vi "Autonomous Independent.vi"() -> ()   [LabVIEW 2015]
doc: "This VI is called when autonomous begins, and will automatically be terminated when autonomous ends. You can carry out timed or sensor driven robot movement independently without needing to return to the caller."
uses:
  <vilib>/Rock Robotics/WPI/SafetyOutput/WPI_SafetyOutputConfigMenu.ctl
  <vilib>/Rock Robotics/Network Tables/NT Read Number.vi
  <vilib>/Rock Robotics/WPI/Utilities/WPI_GetSetVariantRefNum.vi
  <vilib>/Rock Robotics/WPI/Solenoid/Deprecated/WPI_SolenoidGetBool.vi
  <vilib>/Rock Robotics/WPI/Solenoid/Deprecated/WPI_SolenoidSetBool.vi
panel:
  out "Defense Type":dbl=6.0
  in  "Auton_Modes":T1(array[cluster])=[{"Actions"=[{"Action"=enum."Drive", "Effort"=0.55, "Duration"=3.5}, {"Action"=enum."Nothing", "Effort"=0.0, "Duration"=0.0}]}, {"Actions"=[{"Action"=enum."Art Down", "Effort"=0.0, "Duration"=1.0}, {"Action"=enum."Drive", "Effort"=0.75, "Duration"=5.0}, {"Action"=enum."Art Up", "Effort"=0.0, "Duration"=1.0}]}, {"Actions"=[{"Action"=enum."Drive", "Effort"=1.0, "Duration"=3.0}, {"Action"=enum."Art Down", "Effort"=0.0, "Duration"=1.0}, {"Action"=enum."Drive", "Effort"=0.75, "Duration"=3.5}, {"Action"=enum."Art Up", "Effort"=0.0, "Duration"=1.0}]}, {"Actions"=[{"Action"=enum."Shift", "Effort"=0.5, "Duration"=0.0}, {"Action"=enum."Drive", "Effort"=1.0, "Duration"=0.1}, {"Action"=enum."Nothing", "Effort"=0.0, "Duration"=0.1}, {"Action"=enum."Drive", "Effort"=1.0, "Duration"=3.0}]}, {"Actions"=[{"Action"=enum."Shift", "Effort"=0.0, "Duration"=0.0}, {"Action"=enum."Drive", "Effort"=1.0, "Duration"=0.1}, {"Action"=enum."Nothing", "Effort"=0.0, "Duration"=0.1}, {"Action"=enum."Drive", "Effort"=1.0, "Duration"=3.0}]}, {"Actions"=[{"Action"=enum."Shift", "Effort"=0.0, "Duration"=0.0}, {"Action"=enum."Drive", "Effort"=1.0, "Duration"=0.1}, {"Action"=enum."Nothing", "Effort"=0.0, "Duration"=0.1}, {"Action"=enum."Drive", "Effort"=1.0, "Duration"=3.0}]}, {"Actions"=[{"Action"=enum."Drive", "Effort"=0.55, "Duration"=4.0}, {"Action"=enum."Art Down", "Effort"=0.0, "Duration"=1.0}, {"Action"=enum."Drive", "Effort"=-0.5, "Duration"=0.5}, {"Action"=enum."Drive", "Effort"=0.75, "Duration"=1.0}, {"Action"=enum."Art Up", "Effort"=0.0, "Duration"=1.0}, {"Action"=enum."Drive", "Effort"=0.75, "Duration"=3.0}]}, {"Actions"=[{"Action"=enum."Art Down", "Effort"=0.0, "Duration"=0.5}, {"Action"=enum."Drive", "Effort"=0.55, "Duration"=4.25}, {"Action"=enum."Art Up", "Effort"=0.0, "Duration"=0.0}, {"Action"=enum."Nothing", "Effort"=0.0, "Duration"=0.3}, {"Action"=enum."Drive", "Effort"=0.9, "Duration"=2.0}]}, {"Actions"=[{"Action"=enum."Nothing", "Effort"=0.0, "Duration"=0.0}]}]
  # "0 Reach Defense\n1 Low Bar\n2 Rough Terrain\n3 Moat\n4 Rock Wall\n5 Ramparts\n6 Cheval\n7 Portcullis\n8 None"
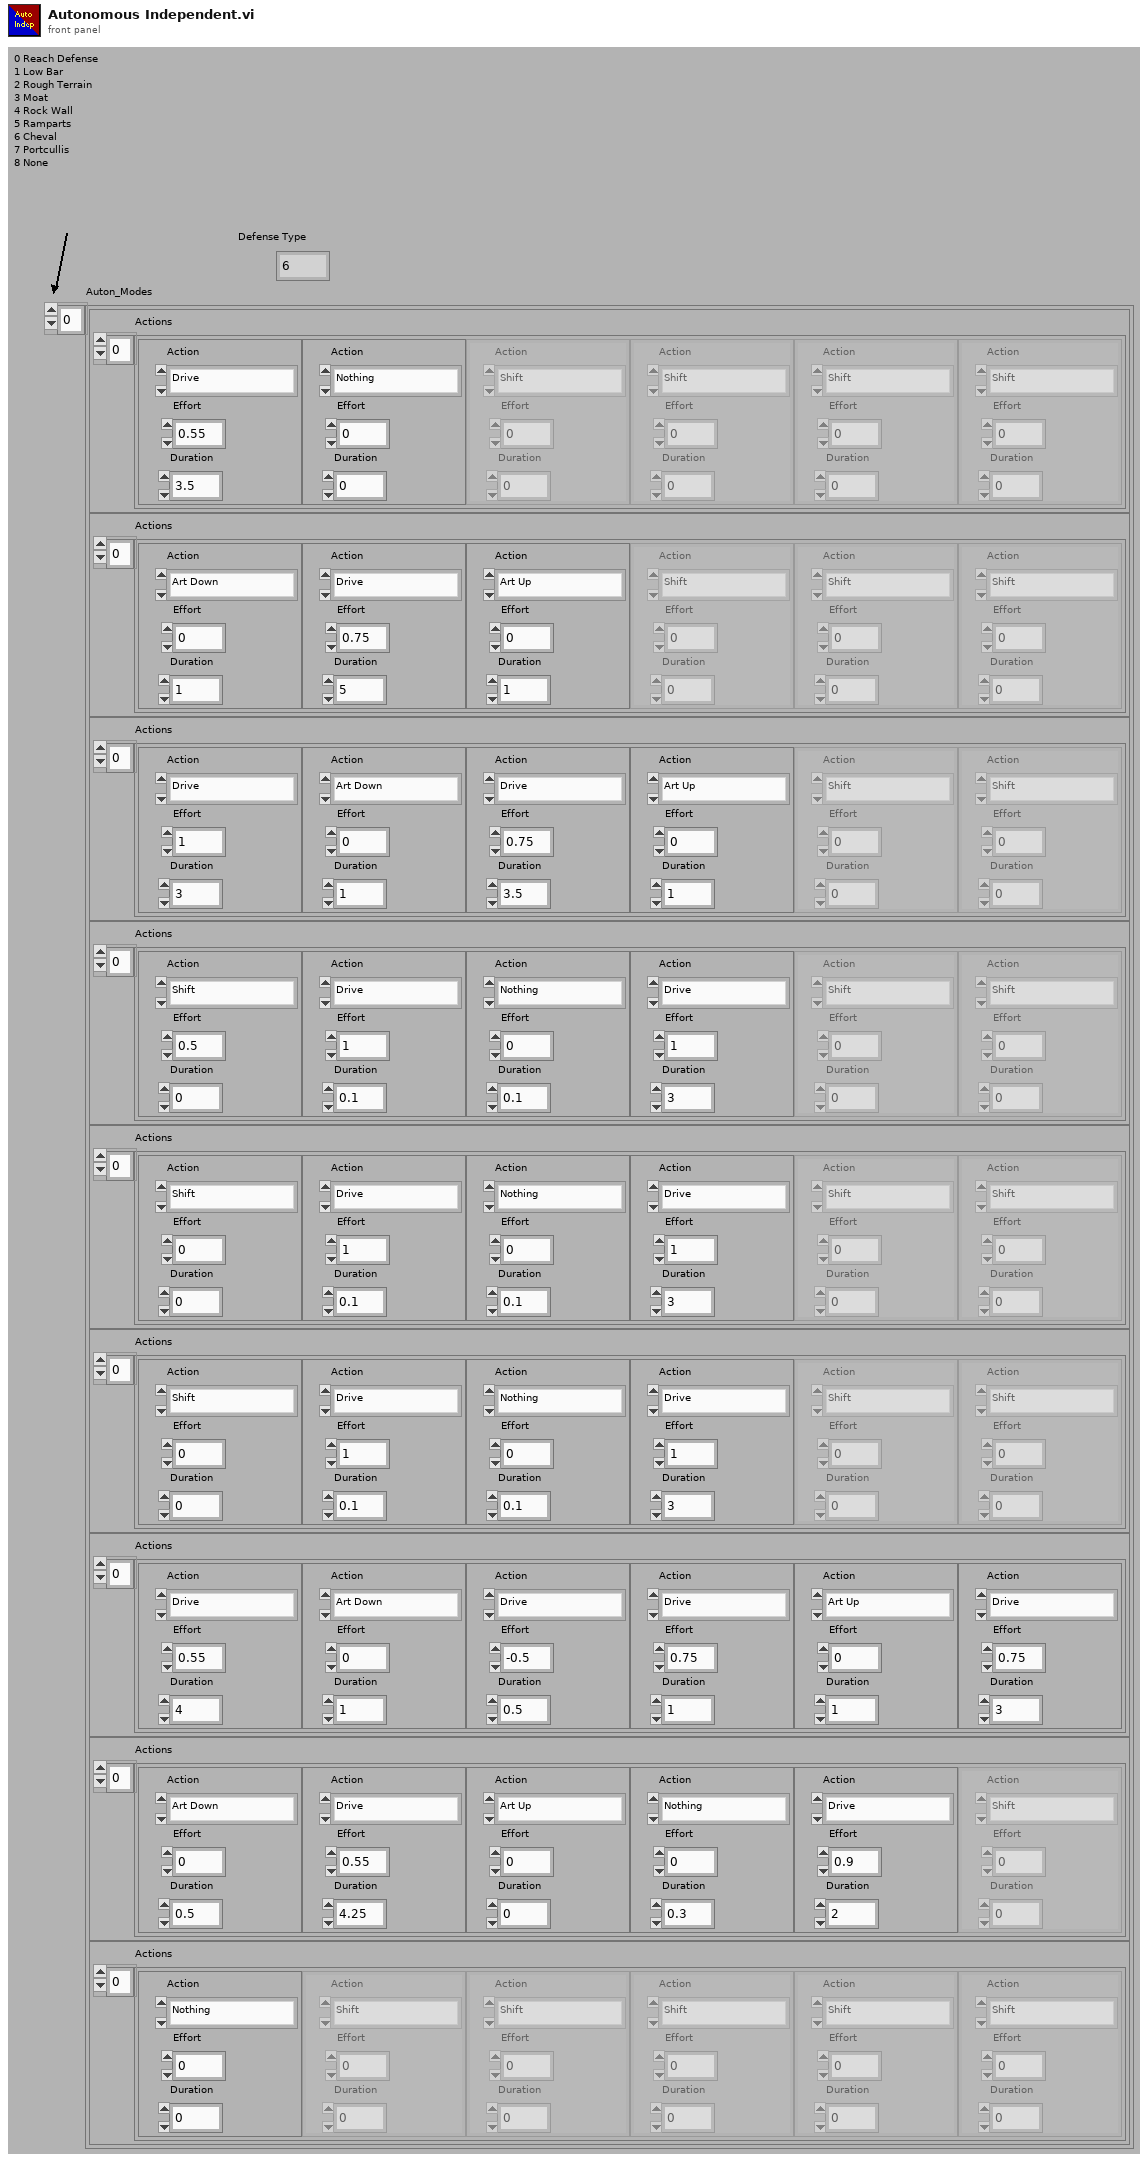
[diagram p1: front panel]
types:
  T1 = cluster{"Actions":cluster{"Action":enum16{"Shift", "Shoot", "Move Articulates", "Nothing", "Drive", "Turn", "Vision Shot", "Art Up", "Art Down", "Test"}, "Effort":dbl, "Duration":dbl}[]}[]
  T2 = cluster{"Actions":cluster{"Action":enum16{"Shift", "Shoot", "Move Articulates", "Nothing", "Drive", "Turn", "Vision Shot", "Art Up", "Art Down", "Test"}, "Effort":dbl, "Duration":dbl}[]}
  T3 = cluster{"Action":enum16{"Shift", "Shoot", "Move Articulates", "Nothing", "Drive", "Turn", "Vision Shot", "Art Up", "Art Down", "Test"}, "Effort":dbl, "Duration":dbl}[]
  T4 = typedef "WPI_SafetyOutputConfigMenu.ctl" = enum16{"Enable", "Disable"}
  T5 = enum16{"Shift", "Shoot", "Move Articulates", "Nothing", "Drive", "Turn", "Vision Shot", "Art Up", "Art Down", "Test"}
  T6 = typedef "WPI_RobotDriveDevRef.ctl" = cluster{"DevStatus":errorcluster, "Motors[]":T7[], "Square Inputs":bool, "Max Output":dbl}
  T7 = typedef "WPI_MotorControlDeviceRef.ctl" = cluster{"DeviceStatus":errorcluster, "Type":T8, "PWM":cluster{"PWM Channel":T9, "DeadBand":T10}, "CAN":cluster{"Device Number":u8, "Control Mode":T11, "Semaphore":T12, "Max Vout":dbl, "TalonSRX Control Mode":T13}, "Invert":bool}
  T8 = typedef "WPI_MotorControlType.ctl" = enum16{"PWM", "CAN", "CANTalonSRX"}
  T9 = typedef "FPGA_DIOPWMChannel.ctl" = enum8{"PWM 0", "PWM 1", "PWM 2", "PWM 3", "PWM 4", "PWM 5", "PWM 6", "PWM 7", "PWM 8", "PWM 9", "PWM MXP 0", "PWM MXP 1", "PWM MXP 2", "PWM MXP 3", "PWM MXP 4", "PWM MXP 5", "PWM MXP 6", "PWM MXP 7", "PWM MXP 8", "PWM MXP 9", "Invalid"}
  T10 = typedef "WPI_PWMDeadband.ctl" = cluster{"Name":string, "maxPositivePwm":i32, "minPositivePwm":i32, "centerPwm":i32, "maxNegativePwm":i32, "minNegativePwm":i32, "angularRange":u16}
  T11 = typedef "WPI_CANJaguar_ControlMode.ctl" = enum8{"Percent VBus", "Current", "Speed", "Position", "Voltage"}
  T12 = typedef "Semaphore RefNum" = refnum<k1>
  T13 = typedef "WPI_CANTalonSRX_APIControlMode.ctl" = enum8{"Percent VBus", "Speed", "Position", "Slave", "Unchanged / Invalid", "Voltage Compensation", "Current", "Motion Profile"}
  T14 = typedef "WPI_SolenoidDevRef.ctl" = cluster{"DevStatus":errorcluster, "Pneumatics Control Module":u8, "Forward Solenoid Channel":T15, "Reverse Solenoid Channel":T15}
  T15 = typedef "WPI_SolenoidChannel.ctl" = enum8{"Solenoid 0", "Solenoid 1", "Solenoid 2", "Solenoid 3", "Solenoid 4", "Solenoid 5", "Solenoid 6", "Solenoid 7", "Invalid"}
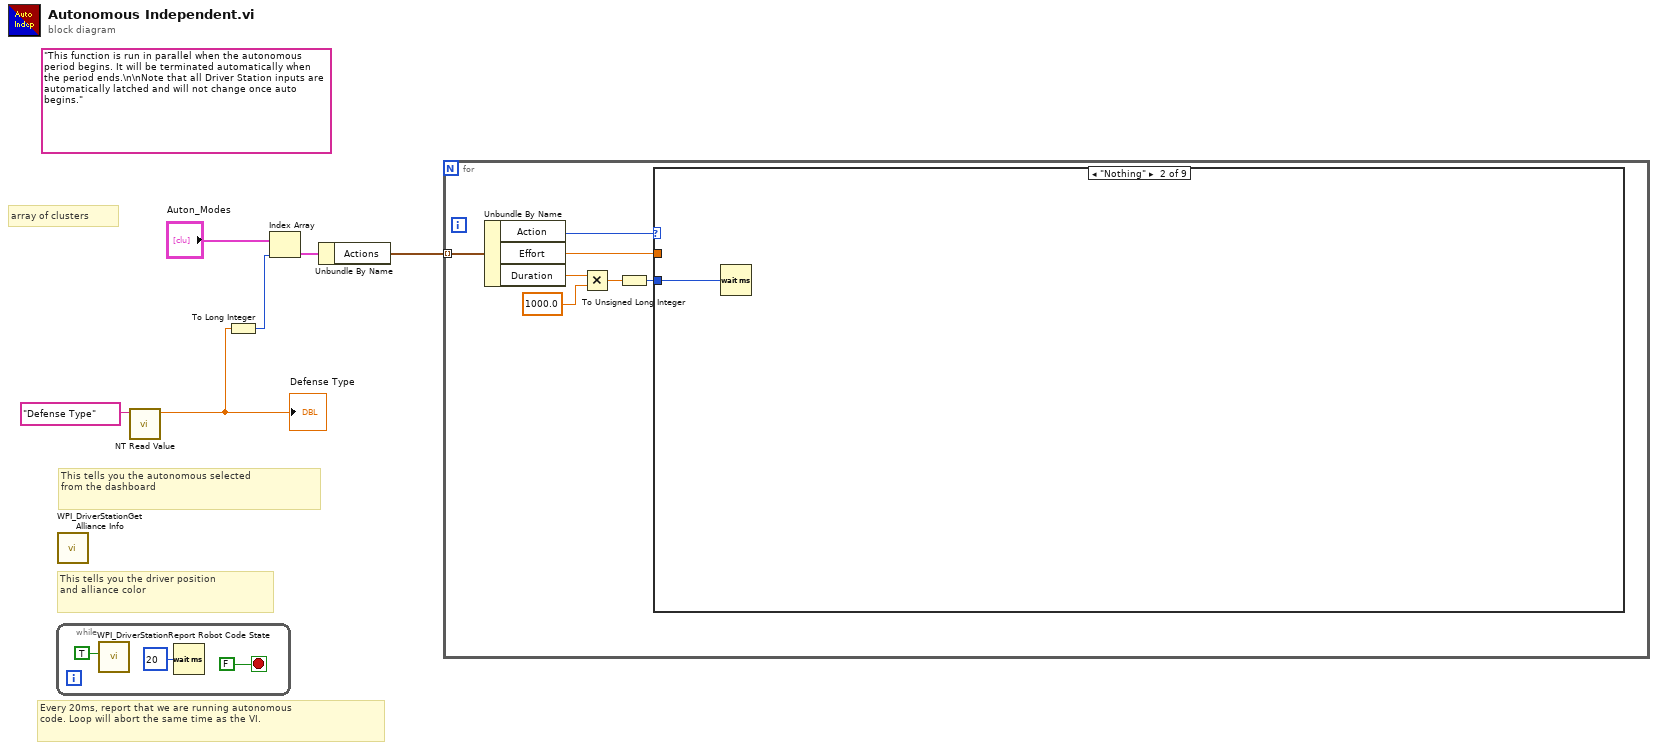
[diagram p0: block diagram]
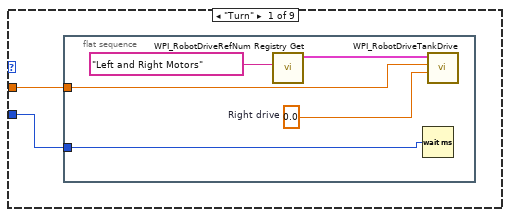
[diagram p2: hidden frame]
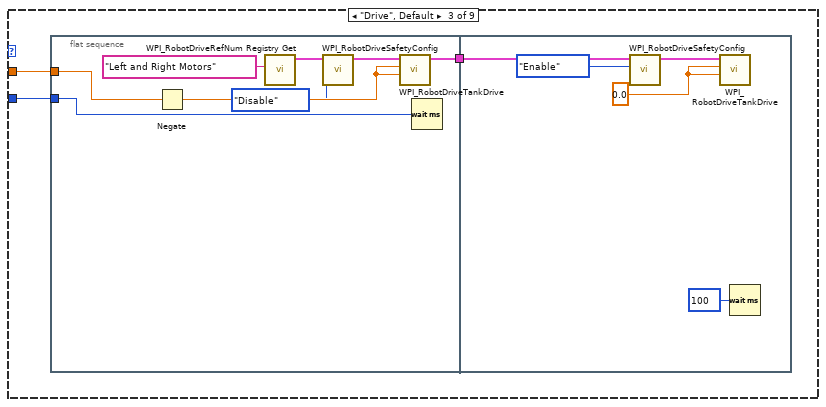
[diagram p3: hidden frame]
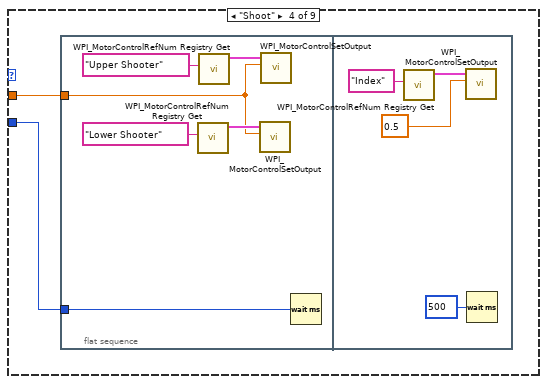
[diagram p4: hidden frame]
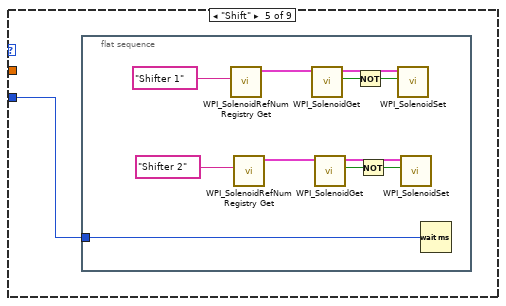
[diagram p5: hidden frame]
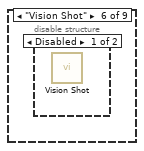
[diagram p6: hidden frame]
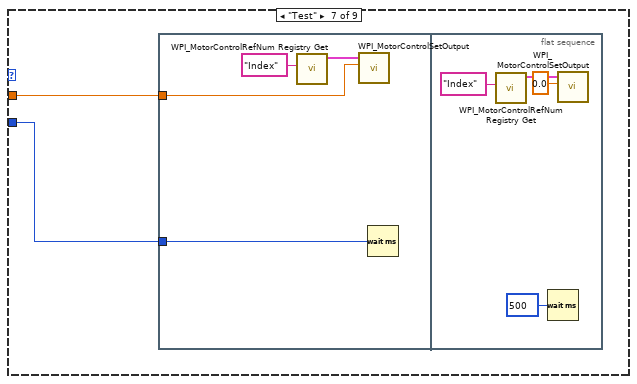
[diagram p8: hidden frame]
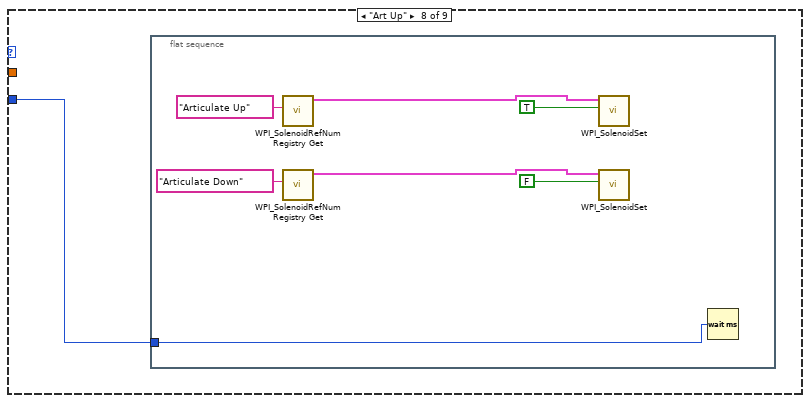
[diagram p9: hidden frame]
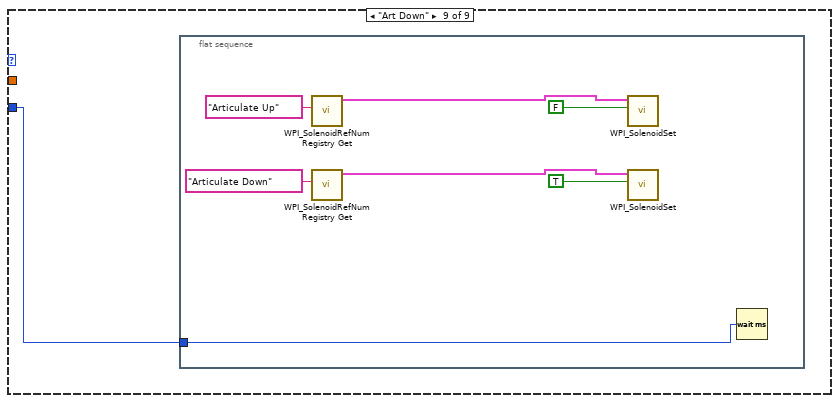
[diagram p10: hidden frame]
diagram:
  (unwired) "This function is run in parallel when the autonomous period begins. It will be terminated automatically when the period ends.\n\nNote that all Driver Station inputs are automatically latched and will not change once auto begins."
  # "This tells you the autonomous selected\nfrom the dashboard"
  # "array of clusters"
  # "Every 20ms, report that we are running autonomous\ncode. Loop will abort the same time as the VI."
  # "This tells you the driver position\nand alliance color"
  n1 = while {
    stop <- FALSE stop-if-true
    n2 = call <vilib>:"WPI_DriverStationReport Robot Code State.vi"("Autonomous"=TRUE) -> ()  [unwired: 10 in, 1 out]
    n3 = Wait (ms)(milliseconds to wait=u32 20) -> ()  [unwired: 1 out]
  }
  n4 = call <vilib>:"WPI_DriverStationGet Alliance Info.vi"() -> ()  [unwired: 12 out]
  n5 = call-poly <vilib>:"NT Read Value.vi"("Name"="Defense Type") -> ("Numeric"=w1:dbl)  [unwired: 9 in, 1 out]
  "Defense Type" <- w1
  n6 = To Long Integer(number=w1) -> (32bit integer=w3:i32)
  n7 = Index Array(array="Auton_Modes", index=w3) -> (element=w5:T2)
  n8 = Unbundle By Name(w5) -> ("Actions"=w6:T3)
  n9 = for {
    tunnel: w6 -> [w16] mode=indexing
    n10 = Unbundle By Name(w16) -> ("Action"=w15:T5, "Effort"=w14:dbl, "Duration"=w13:dbl)
    n11 = Multiply(x=w13, y=1000.0) -> (x*y=w10:dbl)
    n12 = To Unsigned Long Integer(number=w10) -> (unsigned 32bit integer=w11:u32)
    n13 = case shown="\"Nothing\"" w15 {
      tunnel: w14 -> [w18 _ w27 w41 _ _ w66 _ _]
      tunnel: w11 -> [w17 w24 w26 w42 w53 _ w65 w75 w83]
      frame "Turn" {
        n14 = flat-sequence {
          tunnel: w18 -> [w20]
          tunnel: w17 -> [w19]
          frame #0 {
            w22 = 0.0  # Right drive
            n15 = call <vilib>:"WPI_RobotDriveRefNum Registry Get.vi"("refnum name"="Left and Right Motors") -> ("RobotDriveDevRef"=w21:T6)  [unwired: 9 in, 1 out]
            n16 = Wait (ms)(milliseconds to wait=w19) -> ()  [unwired: 1 out]
            n17 = call <vilib>:"WPI_RobotDriveTankDrive.vi"("Right axis value"=w22, "Left axis value"=w20, "RobotDriveDevRef"=w21) -> ()  [unwired: 6 in, 3 out]
          }
        }
      }
      frame "Nothing" {
        n18 = Wait (ms)(milliseconds to wait=w24) -> ()  [unwired: 1 out]
      }
      frame "Drive", Default {
        n19 = flat-sequence {
          tunnel: w27 -> [w33]
          tunnel: w26 -> [w32]
          tunnel: [w30] -> w25
          tunnel: w25 -> [w38]
          frame #0 {
            n20 = Negate(x=w33) -> (-x=w31:dbl)
            n21 = call <vilib>:"WPI_RobotDriveRefNum Registry Get.vi"("refnum name"="Left and Right Motors") -> ("RobotDriveDevRef"=w34:T6)  [unwired: 9 in, 1 out]
            n22 = call <vilib>:"WPI_RobotDriveSafetyConfig.vi"("mode"=WPI_SafetyOutputConfigMenu."Disable", "RobotDriveDevRef"=w34) -> ("RobotDriveDevRef"=w29:T6)  [unwired: 8 in, 1 out]
            n23 = call <vilib>:"WPI_RobotDriveTankDrive.vi"("Right axis value"=w31, "Left axis value"=w31, "RobotDriveDevRef"=w29) -> ("RobotDriveDevRef"=w30:T6)  [unwired: 6 in, 2 out]
            n24 = Wait (ms)(milliseconds to wait=w32) -> ()  [unwired: 1 out]
          }
          frame #1 {
            w40 = 0.0
            n25 = call <vilib>:"WPI_RobotDriveSafetyConfig.vi"("mode"=WPI_SafetyOutputConfigMenu."Enable", "RobotDriveDevRef"=w38) -> ("RobotDriveDevRef"=w37:T6)  [unwired: 8 in, 1 out]
            n26 = call <vilib>:"WPI_RobotDriveTankDrive.vi"("Right axis value"=w40, "Left axis value"=w40, "RobotDriveDevRef"=w37) -> ()  [unwired: 6 in, 3 out]
            n27 = Wait (ms)(milliseconds to wait=u32 100) -> ()  [unwired: 1 out]
          }
        }
      }
      frame "Shoot" {
        n28 = flat-sequence {
          tunnel: w42 -> [w43]
          tunnel: w41 -> [w44]
          frame #0 {
            n29 = call <vilib>:"WPI_MotorControlRefNum Registry Get.vi"("refnum name"="Lower Shooter") -> ("MotorControlDevRef"=w45:T7)  [unwired: 9 in, 1 out]
            n30 = call <vilib>:"WPI_MotorControlRefNum Registry Get.vi"("refnum name"="Upper Shooter") -> ("MotorControlDevRef"=w48:T7)  [unwired: 9 in, 1 out]
            n31 = call <vilib>:"WPI_MotorControlSetOutput.vi"("Output"=w44, "MotorControlDevRef"=w45) -> ()  [unwired: 7 in, 3 out]
            n32 = call <vilib>:"WPI_MotorControlSetOutput.vi"("Output"=w44, "MotorControlDevRef"=w48) -> ()  [unwired: 7 in, 3 out]
            n33 = Wait (ms)(milliseconds to wait=w43) -> ()  [unwired: 1 out]
          }
          frame #1 {
            n34 = call <vilib>:"WPI_MotorControlRefNum Registry Get.vi"("refnum name"="Index") -> ("MotorControlDevRef"=w51:T7)  [unwired: 9 in, 1 out]
            n35 = call <vilib>:"WPI_MotorControlSetOutput.vi"("Output"=0.5, "MotorControlDevRef"=w51) -> ()  [unwired: 7 in, 3 out]
            n36 = Wait (ms)(milliseconds to wait=u32 500) -> ()  [unwired: 1 out]
          }
        }
      }
      frame "Shift" {
        n37 = flat-sequence {
          tunnel: w53 -> [w54]
          frame #0 {
            n38 = call <vilib>:"WPI_SolenoidRefNum Registry Get.vi"("refnum name"="Shifter 1") -> ("SolenoidDevRef"=w64:T14)  [unwired: 9 in, 1 out]
            n39 = call <vilib>:"WPI_SolenoidRefNum Registry Get.vi"("refnum name"="Shifter 2") -> ("SolenoidDevRef"=w55:T14)  [unwired: 9 in, 1 out]
            n40 = call-poly <vilib>:"WPI_SolenoidGet.vi"("SolenoidDevRef"=w64) -> ("Value"=w62:bool, "SolenoidDevRef"=w63:T14)  [unwired: 8 in, 1 out]
            n41 = call-poly <vilib>:"WPI_SolenoidGet.vi"("SolenoidDevRef"=w55) -> ("Value"=w57:bool, "SolenoidDevRef"=w56:T14)  [unwired: 8 in, 1 out]
            n42 = Not(x=w62) -> (.not. x?=w60:bool)
            n43 = Not(x=w57) -> (.not. x?=w59:bool)
            n44 = call-poly <vilib>:"WPI_SolenoidSet.vi"("Value"=w60, "SolenoidDevRef"=w63) -> ()  [unwired: 8 in, 2 out]
            n45 = call-poly <vilib>:"WPI_SolenoidSet.vi"("Value"=w59, "SolenoidDevRef"=w56) -> ()  [unwired: 8 in, 2 out]
            n46 = Wait (ms)(milliseconds to wait=w54) -> ()  [unwired: 1 out]
          }
        }
      }
      frame "Vision Shot" {
        n47 = disable-structure shown="Disabled" {
          frame Disabled {
            n48 = call "Vision Shot.vi"() -> ()  [unwired: 12 in]
          }
          frame Enabled {
          }
        }
      }
      frame "Test" {
        n49 = flat-sequence {
          tunnel: w66 -> [w68]
          tunnel: w65 -> [w67]
          frame #0 {
            n50 = call <vilib>:"WPI_MotorControlRefNum Registry Get.vi"("refnum name"="Index") -> ("MotorControlDevRef"=w70:T7)  [unwired: 9 in, 1 out]
            n51 = call <vilib>:"WPI_MotorControlSetOutput.vi"("Output"=w68, "MotorControlDevRef"=w70) -> ()  [unwired: 7 in, 3 out]
            n52 = Wait (ms)(milliseconds to wait=w67) -> ()  [unwired: 1 out]
          }
          frame #1 {
            n53 = call <vilib>:"WPI_MotorControlRefNum Registry Get.vi"("refnum name"="Index") -> ("MotorControlDevRef"=w73:T7)  [unwired: 9 in, 1 out]
            n54 = Wait (ms)(milliseconds to wait=u32 500) -> ()  [unwired: 1 out]
            n55 = call <vilib>:"WPI_MotorControlSetOutput.vi"("Output"=0.0, "MotorControlDevRef"=w73) -> ()  [unwired: 7 in, 3 out]
          }
        }
      }
      frame "Art Up" {
        n56 = flat-sequence {
          tunnel: w75 -> [w76]
          frame #0 {
            n57 = call <vilib>:"WPI_SolenoidRefNum Registry Get.vi"("refnum name"="Articulate Up") -> ("SolenoidDevRef"=w80:T14)  [unwired: 9 in, 1 out]
            n58 = call <vilib>:"WPI_SolenoidRefNum Registry Get.vi"("refnum name"="Articulate Down") -> ("SolenoidDevRef"=w77:T14)  [unwired: 9 in, 1 out]
            n59 = call-poly <vilib>:"WPI_SolenoidSet.vi"("Value"=TRUE, "SolenoidDevRef"=w80) -> ()  [unwired: 8 in, 2 out]
            n60 = call-poly <vilib>:"WPI_SolenoidSet.vi"("Value"=FALSE, "SolenoidDevRef"=w77) -> ()  [unwired: 8 in, 2 out]
            n61 = Wait (ms)(milliseconds to wait=w76) -> ()  [unwired: 1 out]
          }
        }
      }
      frame "Art Down" {
        n62 = flat-sequence {
          tunnel: w83 -> [w84]
          frame #0 {
            n63 = call <vilib>:"WPI_SolenoidRefNum Registry Get.vi"("refnum name"="Articulate Up") -> ("SolenoidDevRef"=w88:T14)  [unwired: 9 in, 1 out]
            n64 = call <vilib>:"WPI_SolenoidRefNum Registry Get.vi"("refnum name"="Articulate Down") -> ("SolenoidDevRef"=w85:T14)  [unwired: 9 in, 1 out]
            n65 = call-poly <vilib>:"WPI_SolenoidSet.vi"("Value"=FALSE, "SolenoidDevRef"=w88) -> ()  [unwired: 8 in, 2 out]
            n66 = call-poly <vilib>:"WPI_SolenoidSet.vi"("Value"=TRUE, "SolenoidDevRef"=w85) -> ()  [unwired: 8 in, 2 out]
            n67 = Wait (ms)(milliseconds to wait=w84) -> ()  [unwired: 1 out]
          }
        }
      }
    }
  }
